vi "initCAN2.vi"(2 "BaudRate":u32=1000000, 3 "SlotNum":u32, 4 "CAN":cluster{"Interface":refnum<k21>[], "Slot":u32[]}) -> (0 "session write":refnum<k21>, 1 "session read":refnum<k21>)   [LabVIEW 2021]
uses:
  <vilib>/xnet/xnet.llb/XNET Create Session (Frame Input Stream).vi
  <vilib>/xnet/xnet.llb/XNET Create Session (Frame Output Stream).vi
  <resource>/objmgr/xnet.rc
panel:
  out "error out":errorcluster
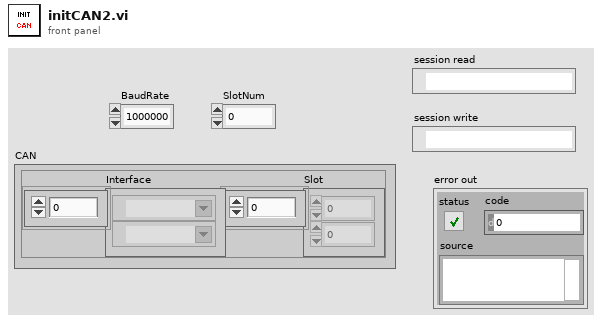
[diagram p1: front panel]
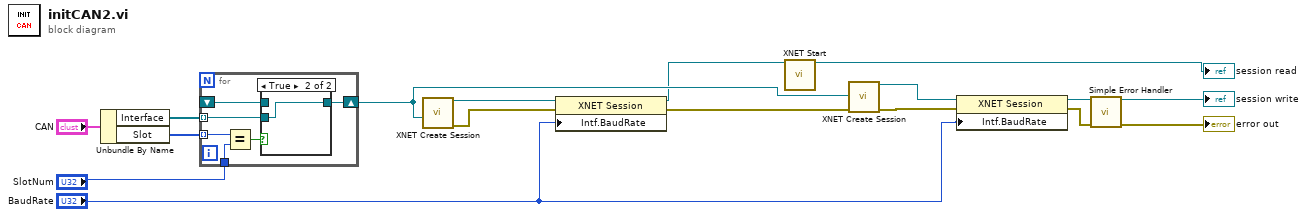
[diagram p0: block diagram]
diagram:
  n1 = Unbundle By Name("CAN") -> ("Interface"=w7:refnum<k21>[], "Slot"=w8:u32[])
  n2 = for {
    tunnel: w8 -> [w22] mode=indexing
    tunnel: w7 -> [w20] mode=indexing
    shift-right: [w19] -> w5
    shift-left: _ -> [w18]
    tunnel: "SlotNum" -> [w17]
    n3 = Equal?(x=w22, y=w17) -> (x = y?=w21:bool)
    n4 = case shown="True" w21 {
      tunnel: w20 -> [_ w24]
      tunnel: [w23 w24] -> w19
      tunnel: w18 -> [w23 _]
      frame False {
      }
      frame True {
      }
    }
  }
  n5 = call-poly <vilib>:"XNET Create Session.vi"("interface"=w5) -> ("session out"=w14:refnum<k21>, "error out"=w15:errorcluster)  [unwired: 2 in, 11 out]
  n6 = property class="XNET Session"(reference=w14, error in=w15, "Intf.BaudRate"="BaudRate") -> (reference out=w2:refnum<k21>, error out=w3:errorcluster)
  n7 = call <vilib>:"XNET Start.vi"("session in"=w2) -> ("session out"=→"session read":refnum<k21>)  [unwired: 13 in, 1 out]
  n8 = call-poly <vilib>:"XNET Create Session.vi"("interface"=w5, "error in (no error)"=w3) -> ("session out"=w16:refnum<k21>, "error out"=w12:errorcluster)  [unwired: 1 in, 11 out]
  n9 = property class="XNET Session"(reference=w16, error in=w12, "Intf.BaudRate"="BaudRate") -> (reference out=→"session write":refnum<k21>, error out=w13:errorcluster)
  n10 = call <vilib>:"Simple Error Handler.vi"("error in (no error)"=w13) -> ("error out"=→"error out":errorcluster)  [unwired: 4 in, 4 out]
